vi "LabvolutionSubmoduleCheck_Global_OnCommand.vi"(10 "Command ID":string, 11 "Object":T1) -> ()   [LabVIEW 2018]
uses:
  <resource>/Framework/Providers/API/ItemRef.ctl
  LabvolutionSubmoduleCheck_File_Action..enum.ctl
panel:
  out "error out":errorcluster
  in  "error in":errorcluster
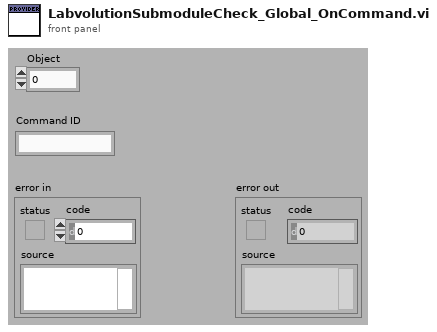
[diagram p1: front panel]
types:
  T1 = typedef "ItemRef.ctl" = u64
  T2 = typedef "LabvolutionSubmoduleCheck_File_Action..enum.ctl" = enum16{"Create", "Remove", "Check"}
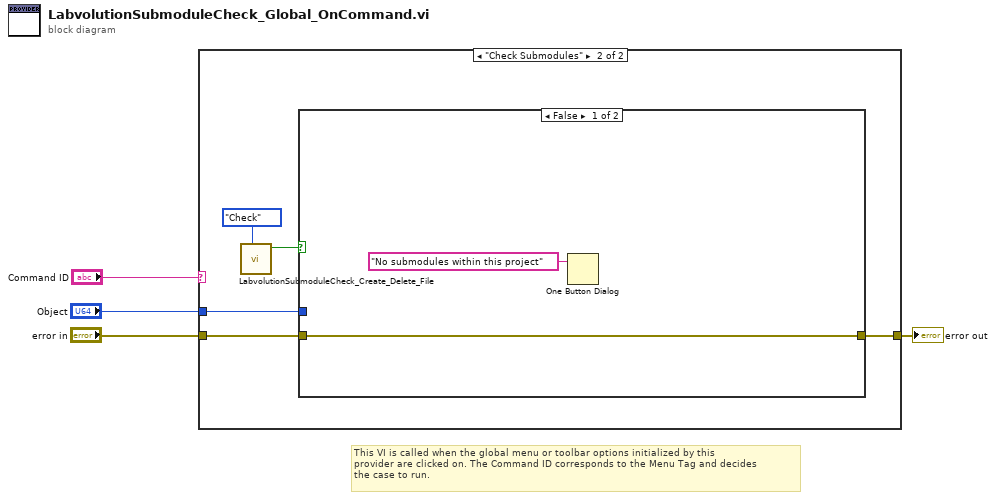
[diagram p0: block diagram]
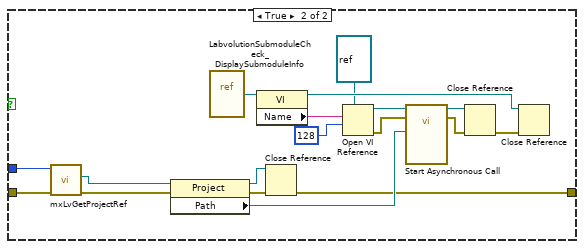
[diagram p3: hidden frame]
diagram:
  # "This VI is called when the global menu or toolbar options initialized by this \nprovider are clicked on. The Command ID corresponds to the Menu Tag and decides\nthe case to run."
  n1 = case shown="\"Check Submodules\"" "Command ID" {
    tunnel: "error in" -> [w5 w9]
    tunnel: [w5 w8] -> w2
    tunnel: "Object" -> [_ w10]
    frame Default {
    }
    frame "Check Submodules" {
      n2 = call "LabvolutionSubmoduleCheck_Create_Delete_File.vi"("Action"=LabvolutionSubmoduleCheck_File_Action..enum."Check") -> ("Submodule Exists"=w7:bool)  [unwired: 9 in, 1 out]
      n3 = case shown="False" w7 {
        tunnel: w10 -> [_ w30]
        tunnel: w9 -> [w12 w28]
        tunnel: [w12 w14] -> w8
        frame False {
          n4 = One Button Dialog(message="No submodules within this project") -> ()  [unwired: 1 in, 1 out]
        }
        frame True {
          n5 = call <resource>:"mxLvGetProjectRef.vi"("error in"=w28, "Item"=w30) -> ("error out"=w29:errorcluster, "Project Refnum"=w27:refnum<vi>)  [unwired: 7 in, 1 out]
          n6 = property class="Project"(reference=w27, error in=w29) -> (reference out=w13:refnum<vi>, error out=w15:errorcluster, "Path"=w16:path)
          n7 = vi-ref "LabvolutionSubmoduleCheck_DisplaySubmoduleInfo.vi"() -> (w17:refnum<vi>)
          n8 = property class="VI"(reference=w17) -> (reference out=w26:refnum<vi>, "Name"=w18:string)  [unwired: 1 in, 1 out]
          n9 = Close Reference(reference=w13, error in (no error)=w15) -> (error out=w14:errorcluster)
          n10 = Open VI Reference(type specifier VI Refnum (for type only)=refnum<vi> refnum, vi path=w18, options=128) -> (vi reference=w21:refnum<vi>, error out=w22:errorcluster)  [unwired: 3 in]
          n11 = call-by-ref "Start Asynchronous Call"(reference=w21, error in=w22, "Project Path"=w16) -> (reference out=w23:refnum<vi>, error out=w24:errorcluster)  [unwired: 11 in]
          n12 = Close Reference(reference=w23, error in (no error)=w24) -> (error out=w25:errorcluster)
          n13 = Close Reference(reference=w26, error in (no error)=w25) -> ()  [unwired: 1 out]
        }
      }
    }
  }
  "error out" <- w2
